vi "Set default graph style.vi"(9 "numero collaudo":i32[](array[numeric]), 10 "Stili default":T2, 11 "PLOT LEGEND in":T1[](array[typedef])=[{"nome plot"="1--18--15--H--Tab1--QH", "colore"=0, "Larghezza linea"=2, "stile linea"=0, "stile punto"=2, "Visibile?"=TRUE, "interpola?"=FALSE, "ordine"=2.0, "ScalaY"=0.0, "Etichetta?"=FALSE, "Freccia? 2"=FALSE, "nome tab?"=FALSE, "Asse Y grafico"="", "Asse X grafico"="", "Grandezza X"="", "Grandezza Y"="", "Collegamento"=0}, {"nome plot"="1--18--15--H--Tab2--QH", "colore"=0, "Larghezza linea"=2, "stile linea"=1, "stile punto"=5, "Visibile?"=TRUE, "interpola?"=FALSE, "ordine"=2.0, "ScalaY"=0.0, "Etichetta?"=FALSE, "Freccia? 2"=FALSE, "nome tab?"=FALSE, "Asse Y grafico"="", "Asse X grafico"="", "Grandezza X"="", "Grandezza Y"="", "Collegamento"=0}, {"nome plot"="CROCE Q1H1", "colore"=16711680, "Larghezza linea"=3, "stile linea"=0, "stile punto"=0, "Visibile?"=FALSE, "interpola?"=FALSE, "ordine"=2.0, "ScalaY"=0.0, "Etichetta?"=FALSE, "Freccia? 2"=FALSE, "nome tab?"=FALSE, "Asse Y grafico"="", "Asse X grafico"="", "Grandezza X"="", "Grandezza Y"="", "Collegamento"=0}, {"nome plot"="CROCE Q2H2", "colore"=16711680, "Larghezza linea"=3, "stile linea"=0, "stile punto"=0, "Visibile?"=FALSE, "interpola?"=FALSE, "ordine"=2.0, "ScalaY"=0.0, "Etichetta?"=FALSE, "Freccia? 2"=FALSE, "nome tab?"=FALSE, "Asse Y grafico"="", "Asse X grafico"="", "Grandezza X"="", "Grandezza Y"="", "Collegamento"=0}] {"Collegamento" items=["TRIFASE"]}) -> (2 "PLOT LEGEND out":T1[](array[typedef])=[{"nome plot"="1--18--15--H--Tab1--QH", "colore"=0, "Larghezza linea"=2, "stile linea"=0, "stile punto"=2, "Visibile?"=TRUE, "interpola?"=FALSE, "ordine"=2.0, "ScalaY"=0.0, "Etichetta?"=FALSE, "Freccia? 2"=FALSE, "nome tab?"=FALSE, "Asse Y grafico"="", "Asse X grafico"="", "Grandezza X"="", "Grandezza Y"="", "Collegamento"=0}, {"nome plot"="1--18--15--H--Tab2--QH", "colore"=0, "Larghezza linea"=2, "stile linea"=1, "stile punto"=5, "Visibile?"=TRUE, "interpola?"=FALSE, "ordine"=2.0, "ScalaY"=0.0, "Etichetta?"=FALSE, "Freccia? 2"=FALSE, "nome tab?"=FALSE, "Asse Y grafico"="", "Asse X grafico"="", "Grandezza X"="", "Grandezza Y"="", "Collegamento"=0}, {"nome plot"="CROCE Q1H1", "colore"=16711680, "Larghezza linea"=3, "stile linea"=0, "stile punto"=0, "Visibile?"=FALSE, "interpola?"=FALSE, "ordine"=2.0, "ScalaY"=0.0, "Etichetta?"=FALSE, "Freccia? 2"=FALSE, "nome tab?"=FALSE, "Asse Y grafico"="", "Asse X grafico"="", "Grandezza X"="", "Grandezza Y"="", "Collegamento"=0}, {"nome plot"="CROCE Q2H2", "colore"=16711680, "Larghezza linea"=3, "stile linea"=0, "stile punto"=0, "Visibile?"=FALSE, "interpola?"=FALSE, "ordine"=2.0, "ScalaY"=0.0, "Etichetta?"=FALSE, "Freccia? 2"=FALSE, "nome tab?"=FALSE, "Asse Y grafico"="", "Asse X grafico"="", "Grandezza X"="", "Grandezza Y"="", "Collegamento"=0}] {"Collegamento" items=["TRIFASE"]})   [LabVIEW 2019]
uses:
  TypeDef/custom plot legend.ctl
panel:
  # "PLOT"
  # "GESTIONE PLOT"
  # "COLLEGAMENTO"
  # "ASSI GRAFICO"
  # "PLOT"
  # "GESTIONE PLOT"
  # "COLLEGAMENTO"
  # "ASSI GRAFICO"
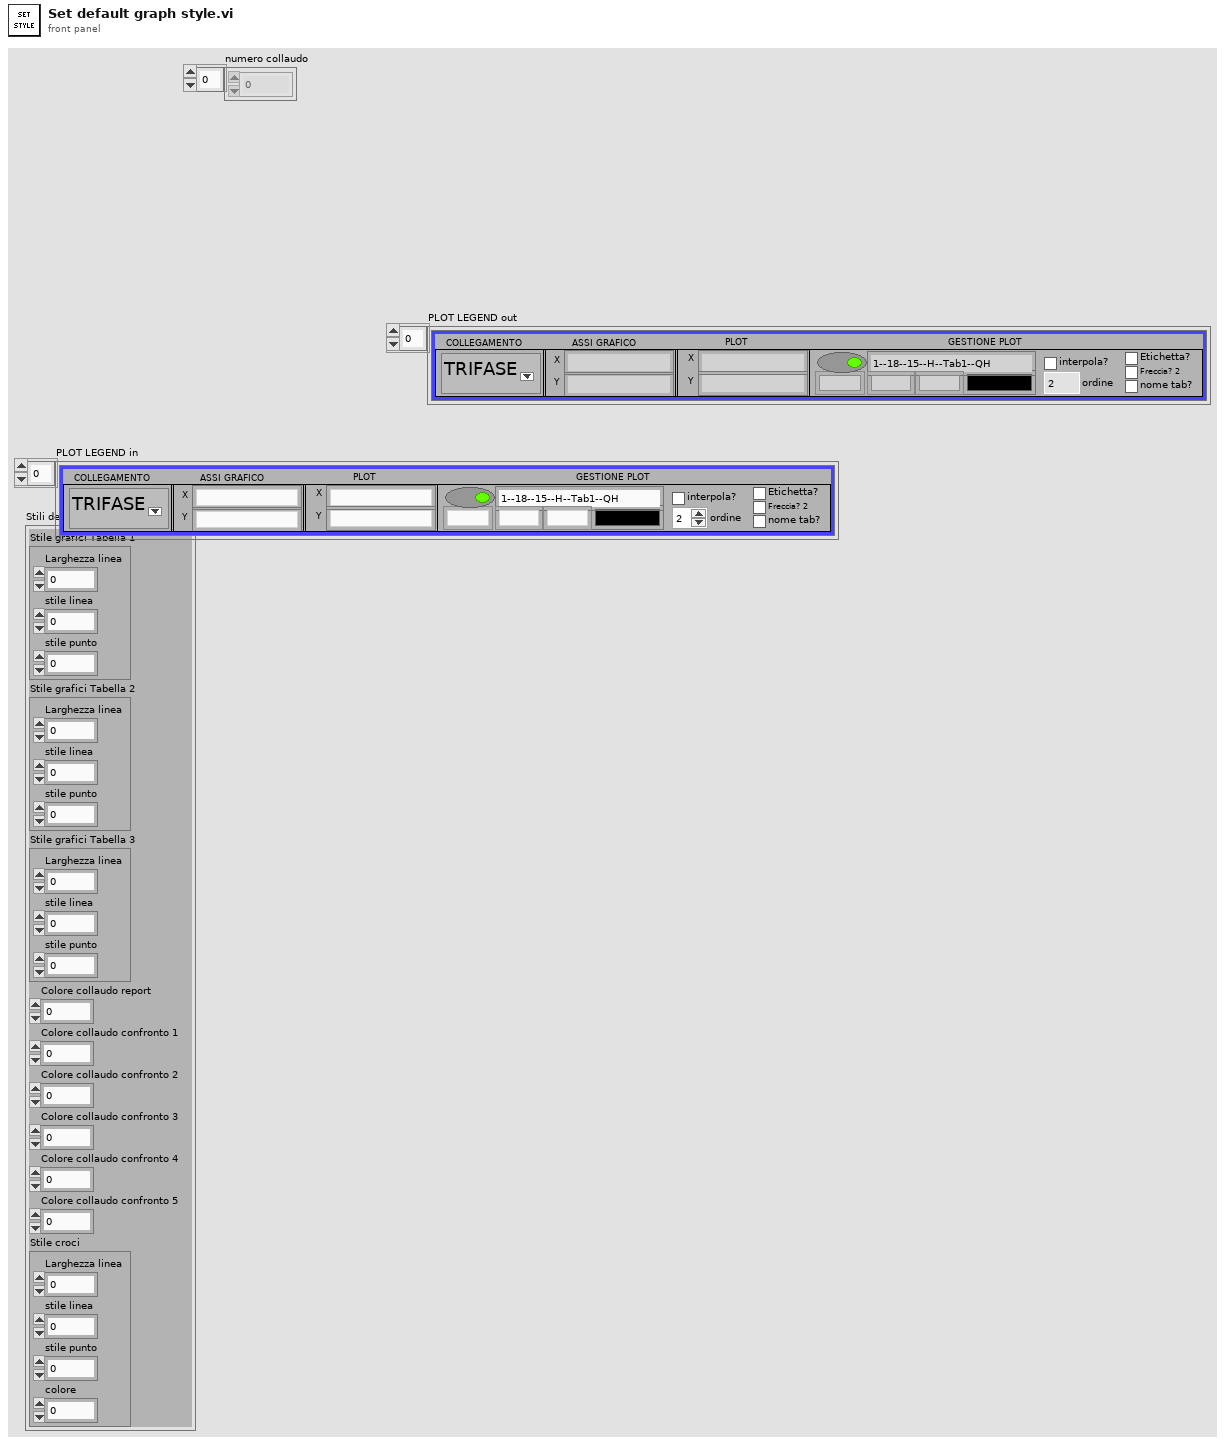
[diagram p1: front panel]
types:
  T1 = typedef "custom plot legend.ctl" = cluster{"nome plot":string, "colore":u32, "Larghezza linea":u16, "stile linea":u16, "stile punto":u16, "Visibile?":bool, "interpola?":bool, "ordine":dbl, "ScalaY":dbl, "Etichetta?":bool, "Freccia? 2":bool, "nome tab?":bool, "Asse Y grafico":string, "Asse X grafico":string, "Grandezza X":string, "Grandezza Y":string, "Collegamento":u16}
  T2 = cluster{"Stile grafici Tabella 1":cluster{"Larghezza linea":u16, "stile linea":u16, "stile punto":u16}, "Stile grafici Tabella 2":cluster{"Larghezza linea":u16, "stile linea":u16, "stile punto":u16}, "Stile grafici Tabella 3":cluster{"Larghezza linea":u16, "stile linea":u16, "stile punto":u16}, "Colore collaudo report":u32, "Colore collaudo confronto 1":u32, "Colore collaudo confronto 2":u32, "Colore collaudo confronto 3":u32, "Colore collaudo confronto 4":u32, "Colore collaudo confronto 5":u32, "Stile croci":cluster{"Larghezza linea":u16, "stile linea":u16, "stile punto":u16, "colore":u32}}
  T3 = cluster{"Larghezza linea":u16, "stile linea":u16, "stile punto":u16, "colore":u32}
  T4 = cluster{"Larghezza linea":u16, "stile linea":u16, "stile punto":u16}
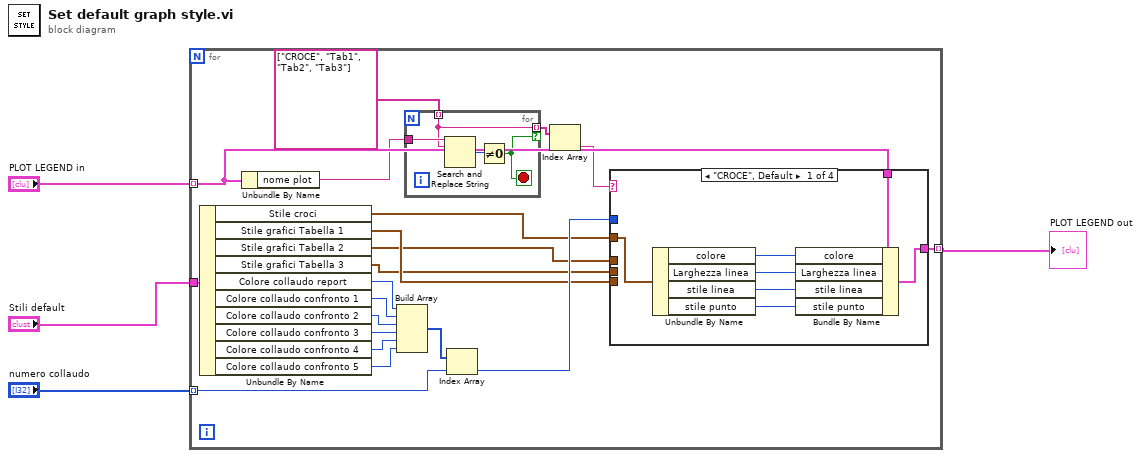
[diagram p0: block diagram]
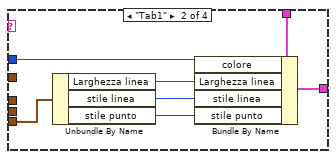
[diagram p2: hidden frame]
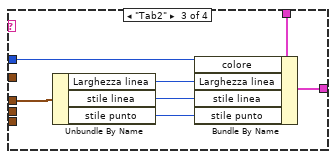
[diagram p3: hidden frame]
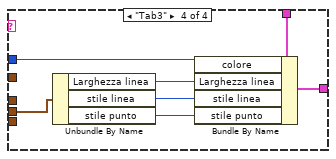
[diagram p4: hidden frame]
diagram:
  n1 = for {
    tunnel: "PLOT LEGEND in" -> [w15] mode=indexing
    tunnel: "Stili default" -> [w24]
    tunnel: "numero collaudo" -> [w16] mode=indexing
    tunnel: [w13] -> w1 mode=indexing
    n2 = Unbundle By Name(w24) -> ("Stile croci"=w5:T3, "Stile grafici Tabella 1"=w8:T4, "Stile grafici Tabella 2"=w7:T4, "Stile grafici Tabella 3"=w6:T4, "Colore collaudo report"=w23:u32, "Colore collaudo confronto 1"=w22:u32, "Colore collaudo confronto 2"=w21:u32, "Colore collaudo confronto 3"=w20:u32, "Colore collaudo confronto 4"=w19:u32, "Colore collaudo confronto 5"=w18:u32)
    n3 = Unbundle By Name(w15) -> ("nome plot"=w12:string)
    n4 = Build Array(w23, w22, w21, w20, w19, w18) -> (w17:u32[])
    n5 = for {
      tunnel: w12 -> [w56]
      tunnel: string[] ["CROCE", "Tab1", "Tab2", "Tab3"] -> [w55] mode=indexing
      tunnel: [w55] -> w10 mode=indexing if=w53
      stop <- w53 stop-if-true
      n6 = Search and Replace String(input string=w56, search string=w55) -> (number of replacements=w54:i32)  [unwired: 6 in, 3 out]
      n7 = Not Equal To 0?(x=w54) -> (x != 0?=w53:bool)
    }
    n8 = Index Array(array=w17, index=w16) -> (element=w14:u32)
    n9 = Index Array(array=w10) -> (element=w9:string)  [unwired: 1 in]
    n10 = case shown="\"CROCE\", Default" w9 {
      tunnel: w15 -> [w31 w38 w45 w52]
      tunnel: w14 -> [_ w37 w44 w51]
      tunnel: [w30 w36 w43 w50] -> w13
      tunnel: w8 -> [_ w35 _ _]
      tunnel: w7 -> [_ _ w39 _]
      tunnel: w6 -> [_ _ _ w46]
      tunnel: w5 -> [w29 _ _ _]
      frame "CROCE", Default {
        n11 = Unbundle By Name(w29) -> ("colore"=w28:u32, "Larghezza linea"=w25:u16, "stile linea"=w26:u16, "stile punto"=w27:u16)
        n12 = Bundle By Name(cluster=w31, "colore"=w28, "Larghezza linea"=w25, "stile linea"=w26, "stile punto"=w27) -> (w30:T1)
      }
      frame "Tab1" {
        n13 = Unbundle By Name(w35) -> ("Larghezza linea"=w34:u16, "stile linea"=w33:u16, "stile punto"=w32:u16)
        n14 = Bundle By Name(cluster=w38, "colore"=w37, "Larghezza linea"=w34, "stile linea"=w33, "stile punto"=w32) -> (w36:T1)
      }
      frame "Tab2" {
        n15 = Unbundle By Name(w39) -> ("Larghezza linea"=w42:u16, "stile linea"=w41:u16, "stile punto"=w40:u16)
        n16 = Bundle By Name(cluster=w45, "colore"=w44, "Larghezza linea"=w42, "stile linea"=w41, "stile punto"=w40) -> (w43:T1)
      }
      frame "Tab3" {
        n17 = Unbundle By Name(w46) -> ("Larghezza linea"=w49:u16, "stile linea"=w48:u16, "stile punto"=w47:u16)
        n18 = Bundle By Name(cluster=w52, "colore"=w51, "Larghezza linea"=w49, "stile linea"=w48, "stile punto"=w47) -> (w50:T1)
      }
    }
  }
  "PLOT LEGEND out" <- w1
